vi "GRAFICA CURVA XY.vi"(9 "Y INDEX":i32, 10 "X INDEX":i32, 11 "Curva 1":string[][](array[string])) -> (3 "Cluster":cluster{"X":dbl[], "Y":dbl[]})   [LabVIEW 2019]
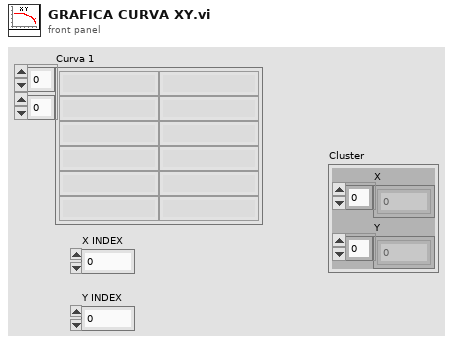
[diagram p1: front panel]
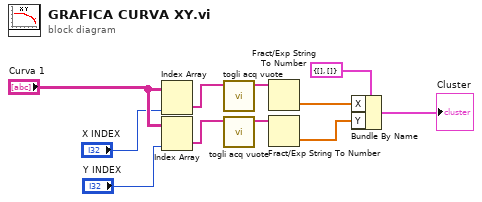
[diagram p0: block diagram]
diagram:
  n1 = Index Array(array="Curva 1", index (col)="X INDEX") -> (element=w1:string[])  [unwired: 1 in]
  n2 = Index Array(array="Curva 1", index (col)="Y INDEX") -> (element=w5:string[])  [unwired: 1 in]
  n3 = call "togli acq vuote.vi"("Q"=w1) -> ("Array"=w2:string[])  [unwired: 10 in]
  n4 = call "togli acq vuote.vi"("Q"=w5) -> ("Array"=w4:string[])  [unwired: 10 in]
  n5 = Fract/Exp String To Number(string=w2) -> (number=w10:dbl[])  [unwired: 3 in, 1 out]
  n6 = Fract/Exp String To Number(string=w4) -> (number=w7:dbl[])  [unwired: 3 in, 1 out]
  n7 = Bundle By Name(cluster=cluster{"X":dbl[], "Y":dbl[]} {"X"=[], "Y"=[]}, "X"=w10, "Y"=w7) -> (→"Cluster":cluster{"X":dbl[], "Y":dbl[]})
